vi "testReadFile.vi"(8 "error in (no error)":errorcluster) -> (0 "error out":errorcluster)   [LabVIEW 2016]
doc: "Test to read the configuration file by line."
uses:
  <vilib>/addons/_JKI Toolkits/Caraya/classes/Assert/Assert.lvclass
  <vilib>/addons/_JKI Toolkits/Caraya/classes/Test/Test.lvclass
  MatOper/MatOper.lvclass
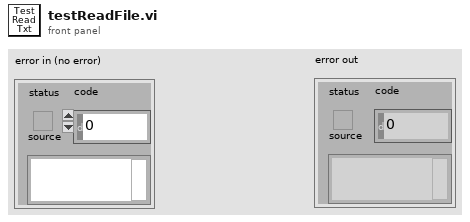
[diagram p1: front panel]
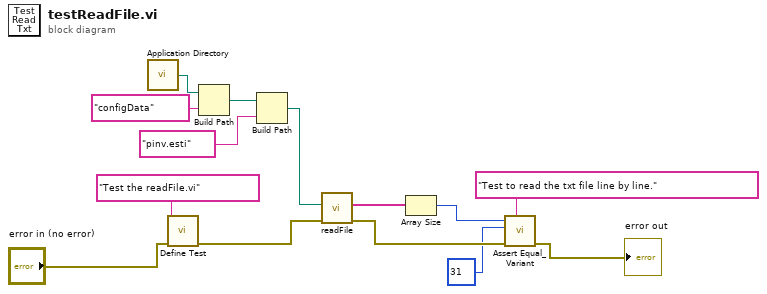
[diagram p0: block diagram]
diagram:
  n1 = call <vilib>:"Application Directory.vi"() -> ("Application Directory"=w5:path)
  n2 = call <vilib>:"Define Test.vi"("error in (no error)"="error in (no error)", "Label (VI Title)"="Test the readFile.vi") -> ("error out"=w10:errorcluster)  [unwired: 9 in]
  n3 = Build Path(base path=w5, name or relative path="configData") -> (appended path=w3:path)
  n4 = Build Path(base path=w3, name or relative path="pinv.esti") -> (appended path=w1:path)
  n5 = call "readFile.vi"("error in (no error)"=w10, "Path"=w1) -> ("error out"=w9:errorcluster, "Array"=w8:string[])  [unwired: 7 in, 1 out]
  n6 = Array Size(array=w8) -> (size(s)=w7:i32)
  n7 = call <vilib>:"Assert Equal_Variant.vi"("Label"="Test to read the txt file line by line.", "error in (no error)"=w9, "Y"=31, "X"=w7) -> ("error out"=→"error out":errorcluster)  [unwired: 7 in]
